vi "FPGA Initialize Session.vi"(4 "max num IRQs":i32=1, 6 "Names of Registers":T1, 7 "Run?":T2, 8 "error in (no error)":errorcluster, 9 "FPGA Resource":string="RIO0", 10 "Bitfile Path":path, 11 "FPGA Interface Base In":refnum<class "FPGA Interface Base.lvclass">) -> (0 "error out":errorcluster, 3 "FPGA Interface Base Out":refnum<class "FPGA Interface Base.lvclass">)   [LabVIEW 2010, in "FPGA Interface Base.lvclass"]
uses:
  <userlib>/_FPGA Interface Advanced Tools/FPGA Interface Base/FPGA Interface Base.lvclass
  <userlib>/_FPGA Interface Advanced Tools/FPGA Interface Wrapper/TypeDefs/Open Attribute.ctl
  <userlib>/_FPGA Interface Advanced Tools/FPGA Interface Base/TypeDefs/FPGA Register Names.ctl
  <userlib>/_FPGA Interface Advanced Tools/FPGA Interface Base/TypeDefs/FPGA Session Data.ctl
  <userlib>/_FPGA Interface Advanced Tools/FPGA Bitfile Utility/TypeDefs/Scalar Register Set.ctl
  <userlib>/_FPGA Interface Advanced Tools/FPGA Bitfile Utility/TypeDefs/Scalar Register.ctl
  <userlib>/_FPGA Interface Advanced Tools/FPGA Bitfile Utility/TypeDefs/Array Register Set.ctl
  <userlib>/_FPGA Interface Advanced Tools/FPGA Bitfile Utility/TypeDefs/Array Register.ctl
  <userlib>/_FPGA Interface Advanced Tools/FPGA Bitfile Utility/TypeDefs/FIFO Channel Set.ctl
  <userlib>/_FPGA Interface Advanced Tools/FPGA Bitfile Utility/TypeDefs/FIFO Channel.ctl
  <userlib>/_FPGA Interface Advanced Tools/FPGA Interface Base/FPGA Interface Base.lvclass/FPGA Interface Base.ctl
  <vilib>/rvi/Utilities/XML/nirviXML_GetValue.vi
  <vilib>/rvi/Utilities/XML/nirviXML_GetValue_String.vi
  <vilib>/Utility/error.llb/Error Cluster From Error Code.vi
  <userlib>/_FPGA Interface Advanced Tools/FPGA Bitfile Utility/FPGA Bitfile Utility.lvlib
  <userlib>/_FPGA Interface Advanced Tools/FPGA Interface Wrapper/FPGA Interface Wrapper.lvlib
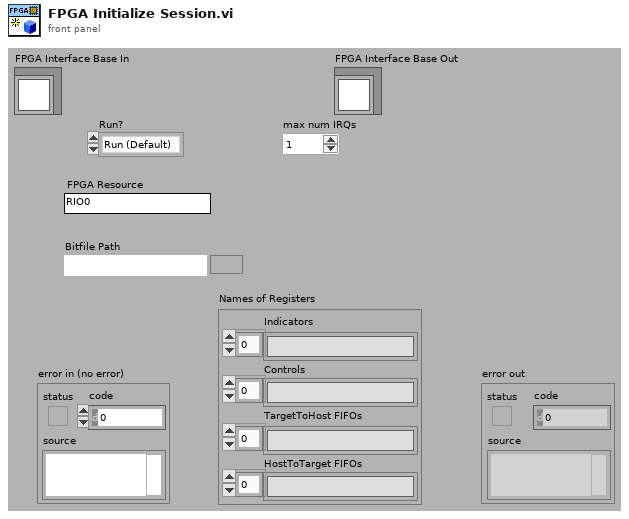
[diagram p1: front panel]
types:
  T1 = typedef "FPGA Interface Base.lvclass/FPGA Register Names.ctl" = cluster{"Indicators":string[], "Controls":string[], "TargetToHost FIFOs":string[], "HostToTarget FIFOs":string[]}
  T2 = typedef "FPGA Interface Wrapper.lvlib/Open Attribute.ctl" = enum32{"Run (Default)", "No Run"}
  T3 = typedef "FPGA Interface Base.lvclass/FPGA Session Data.ctl" = cluster{"Session Out":u32, "Indicator Scalars":T4, "Indicator Arrays":T6, "Control Scalars":T4, "Control Arrays":T6, "TargetToHost FIFO Channels":T8, "HostToTarget FIFO Channels":T8, "All FIFOs":T9[], "IRQ Context Queue":refnum<queue>}
  T4 = typedef "FPGA Bitfile Utility.lvlib/Scalar Register Set.ctl" = cluster{"Boolean":T5[], "I8":T5[], "I16":T5[], "I32":T5[], "I64":T5[], "U8":T5[], "U16":T5[], "U32":T5[], "U64":T5[]}
  T5 = typedef "FPGA Bitfile Utility.lvlib/Scalar Register.ctl" = cluster{"Address":u32, "Name":string}
  T6 = typedef "FPGA Bitfile Utility.lvlib/Array Register Set.ctl" = cluster{"Boolean":T7[], "I8":T7[], "I16":T7[], "I32":T7[], "I64":T7[], "U8":T7[], "U16":T7[], "U32":T7[], "U64":T7[]}
  T7 = typedef "FPGA Bitfile Utility.lvlib/Array Register.ctl" = cluster{"Address":u32, "Num Elements":u32, "Name":string}
  T8 = typedef "FPGA Bitfile Utility.lvlib/FIFO Channel Set.ctl" = cluster{"Boolean":T9[], "I8":T9[], "I16":T9[], "I32":T9[], "I64":T9[], "U8":T9[], "U16":T9[], "U32":T9[], "U64":T9[]}
  T9 = typedef "FPGA Bitfile Utility.lvlib/FIFO Channel.ctl" = cluster{"Physical Channel":u32, "Name":string}
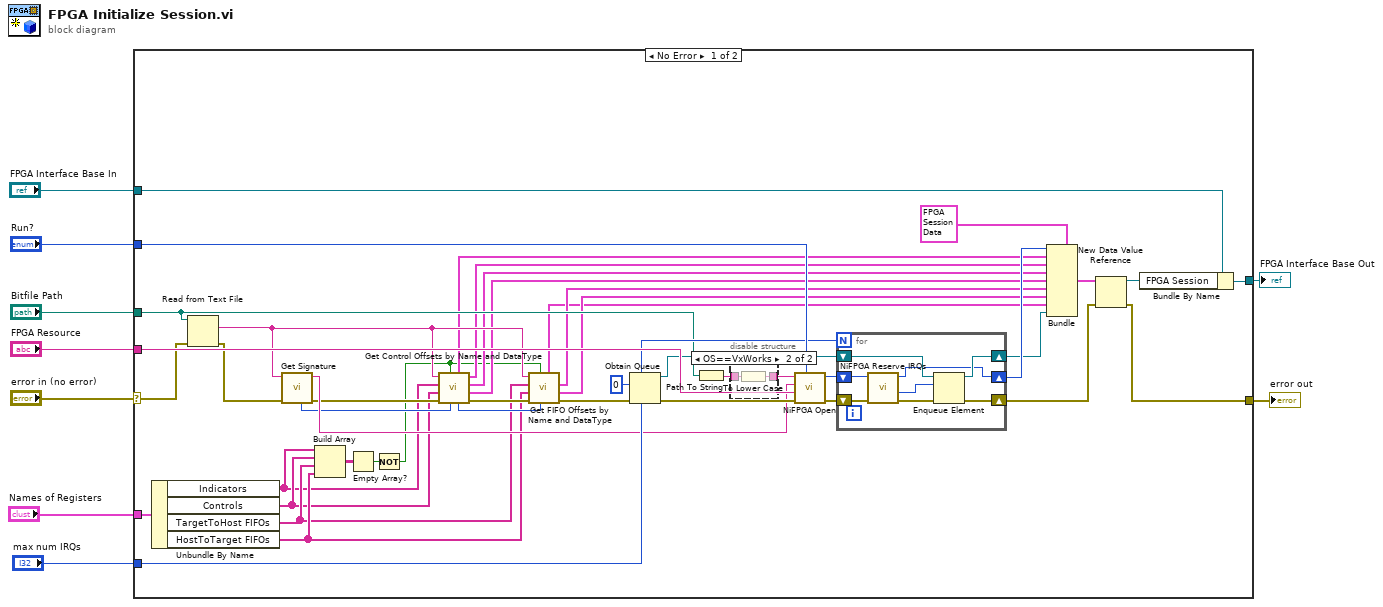
[diagram p0: block diagram]
diagram:
  n1 = case shown="No Error" "error in (no error)" {
    selector: "error in (no error)" -> [w47 w66]
    tunnel: "FPGA Resource" -> [w53 _]
    tunnel: "Bitfile Path" -> [w48 _]
    tunnel: "Names of Registers" -> [w52 _]
    tunnel: "Run?" -> [w51 _]
    tunnel: [w50 w66] -> w4
    tunnel: [w20 w65] -> w2
    tunnel: "max num IRQs" -> [w49 _]
    tunnel: "FPGA Interface Base In" -> [w19 w65]
    frame No Error {
      n2 = Unbundle By Name(w52) -> ("Indicators"=w14:string[], "Controls"=w15:string[], "TargetToHost FIFOs"=w16:string[], "HostToTarget FIFOs"=w17:string[])
      n3 = Read from Text File(file (use dialog)=w48, error in=w47) -> (text=w35:string, error out=w34:errorcluster)  [unwired: 4 out]
      n4 = call <userlib>:"Get Signature.vi"("error in (no error)"=w34, "bitfile xml in"=w35) -> ("error out"=w33:errorcluster, "Bitfile Signature"=w37:string, "offset past EndTag"=w32:i32)  [unwired: 7 in]
      n5 = Build Array(w14, w15, w16, w17) -> (w18:string[][])
      n6 = Empty Array?(array=w18) -> (empty?=w13:bool)
      n7 = Not(x=w13) -> (.not. x?=w12:bool)
      n8 = call <userlib>:"Get Control Offsets by Name and DataType.vi"("offset"=w32, "User Specified?"=w12, "error in"=w33, "Controls"=w15, "Indicators"=w14, "bitfile xml in"=w35) -> ("error out"=w46:errorcluster, "Control Arrays"=w27:T6, "Control Scalars"=w28:T4, "Indicator Arrays"=w29:T6, "offset past EndTag"=w31:i32, "Indicator Scalars"=w30:T4)
      n9 = call <userlib>:"Get FIFO Offsets by Name and DataType.vi"("offset"=w31, "User Specified?"=w12, "error in"=w46, "HostToTarget FIFOs"=w17, "TargetToHost FIFOs"=w16, "bitfile xml in"=w35) -> ("error out"=w36:errorcluster, "HostToTarget"=w26:T8, "TargetToHost"=w25:T8, "All FIFOs"=w23:T9[])  [unwired: 1 in, 1 out]
      n10 = Obtain Queue(max queue size (-1, unlimited)=w49, element data type=u32 0 ("Context"), error in (no error)=w36) -> (queue out=w41:refnum<queue>, error out=w43:errorcluster)  [unwired: 2 in, 1 out]
      n11 = Path To String(path=w48) -> (string=w11:string)
      n12 = disable-structure shown="OS==VxWorks" {
        disable-tunnel: w11 -> [w54 w56]
        disable-tunnel: [w54 w55] -> w10
        frame condition #0 (active) {
        }
        frame condition #1 {
          n13 = To Lower Case(string=w56) -> (all lower case string=w55:string)
        }
      }
      n14 = call <userlib>:"NiFPGA Open.vi"("Attribute"=w51, "error in (no error)"=w43, "Resource"=w53, "Signature"=w37, "Bitfile"=w10) -> ("error out"=w42:errorcluster, "Session Out"=w38:u32)  [unwired: 5 in]
      n15 = for {
        N: w49 -> [_]
        shift-right: [w60] -> w39
        shift-left: w42 -> [w59]
        shift-right: [w58] -> w24
        shift-left: w41 -> [w62]
        shift-right: [w57] -> w40
        shift-left: w38 -> [w64]
        n16 = call <userlib>:"NiFPGA Reserve IRQs.vi"("error in (no error)"=w59, "Session In"=w64) -> ("error out"=w63:errorcluster, "Context"=w61:u32, "Session Out"=w57:u32)  [unwired: 7 in]
        n17 = Enqueue Element(queue=w62, element=w61, error in (no error)=w63) -> (queue out=w58:refnum<queue>, error out=w60:errorcluster)  [unwired: 1 in, 1 out]
      }
      n18 = Bundle(cluster=T3 {"Session Out"=0, "Indicator Scalars"={"Boolean"=[], "I8"=[], "I16"=[], "I32"=[], "I64"=[], "U8"=[], "U16"=[], "U32"=[], "U64"=[]}, "Indicator Arrays"={"Boolean"=[], "I8"=[], "I16"=[], "I32"=[], "I64"=[], "U8"=[], "U16"=[], "U32"=[], "U64"=[]}, "Control Scalars"={"Boolean"=[], "I8"=[], "I16"=[], "I32"=[], "I64"=[], "U8"=[], "U16"=[], "U32"=[], "U64"=[]}, "Control Arrays"={"Boolean"=[], "I8"=[], "I16"=[], "I32"=[], "I64"=[], "U8"=[], "U16"=[], "U32"=[], "U64"=[]}, "TargetToHost FIFO Channels"={"Boolean"=[], "I8"=[], "I16"=[], "I32"=[], "I64"=[], "U8"=[], "U16"=[], "U32"=[], "U64"=[]}, "HostToTarget FIFO Channels"={"Boolean"=[], "I8"=[], "I16"=[], "I32"=[], "I64"=[], "U8"=[], "U16"=[], "U32"=[], "U64"=[]}, "All FIFOs"=[], "IRQ Context Queue"=refnum} ("FPGA Session Data"), "Session Out"=w40, "Indicator Scalars"=w30, "Indicator Arrays"=w29, "Control Scalars"=w28, "Control Arrays"=w27, "TargetToHost FIFO Channels"=w25, "HostToTarget FIFO Channels"=w26, "All FIFOs"=w23, "IRQ Context Queue"=w24) -> (w45:T3)
      n19 = New Data Value Reference(data value=w45, error in=w39) -> (data value reference=w21:refnum<data-value>, error out=w50:errorcluster)
      n20 = Bundle By Name(cluster=w19, "FPGA Session"=w21) -> (w20:refnum<class "FPGA Interface Base.lvclass">)
    }
    frame Error {
    }
  }
  "error out" <- w4
  "FPGA Interface Base Out" <- w2
